vi "Close Module.vi"(8 "error in (no error)":errorcluster, 11 "Module Admin in":refnum<class "Delacor_lib_QMH_Module Admin.lvclass">) -> (0 "error out":errorcluster, 1 "External Launch":bool, 3 "Module Admin out":refnum<class "Delacor_lib_QMH_Module Admin.lvclass">)   [LabVIEW 2020, in "Numpad.lvlib"]
doc: "Destroy the Broadcast Events and Request Events. Reset flags stored in Module Admin class.\n_____\nBased on Delacor QMH Project Template 5.0.0.82."
uses:
  Numpad.lvlib
  <vilib>/Delacor/Delacor QMH/Libraries/Module Admin_class/Delacor_lib_QMH_Module Admin.lvclass
  <vilib>/Delacor/Delacor QMH/Libraries/Module Admin_class/Delacor_lib_QMH_Module Admin.lvclass/Delacor_lib_QMH_Module Admin.ctl
  <vilib>/Delacor/Delacor QMH/Libraries/Module Admin_class/Delacor_lib_QMH_Get External Launch.vi
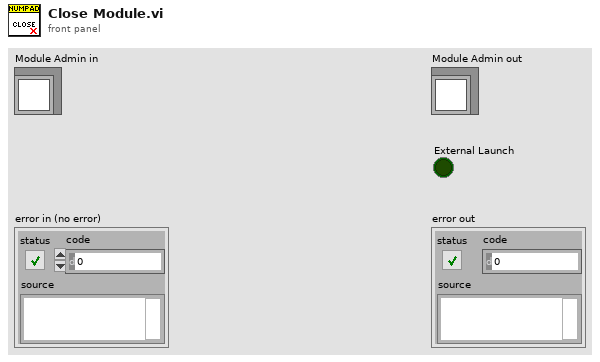
[diagram p1: front panel]
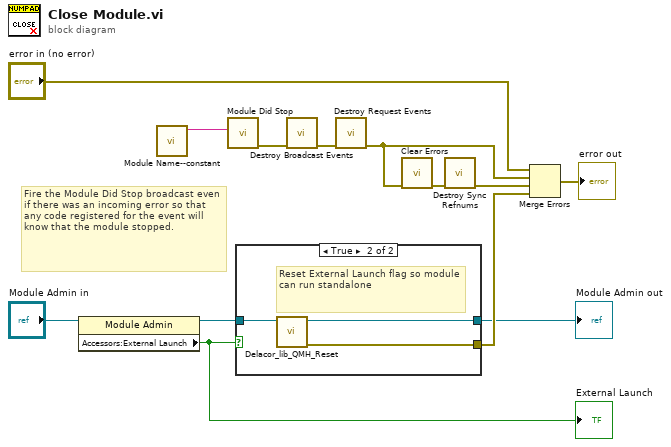
[diagram p0: block diagram]
diagram:
  # "Fire the Module Did Stop broadcast even if there was an incoming error so that any code registered for the event will know that the module stopped."
  n1 = property class="Module Admin"(reference="Module Admin in") -> (reference out=w11:refnum<class "Delacor_lib_QMH_Module Admin.lvclass">, "Accessors:External Launch"=w8:bool)  [unwired: 1 in, 1 out]
  "External Launch" <- w8
  n2 = call "Module Name--constant.vi"() -> ("Module Name"=w6:string)  [unwired: 11 in]
  n3 = call "Module Did Stop.vi"("Origin"=w6) -> ("error out"=w5:errorcluster)  [unwired: 10 in]
  n4 = case shown="True" w8 {
    tunnel: w11 -> [w14 w17]
    tunnel: [w14 w16] -> w9
    tunnel: [_ w15] -> w13
    frame False {
    }
    frame True {
      # "Reset External Launch flag so module can run standalone"
      n5 = call-dynamic "Delacor_lib_QMH_Reset.vi"("Mod Admin in"=w17) -> ("error out"=w15:errorcluster, "Mod Admin out"=w16:refnum<class "Delacor_lib_QMH_Module Admin.lvclass">)  [unwired: 9 in]
    }
  }
  "Module Admin out" <- w9
  n6 = call "Destroy Broadcast Events.vi"("error in (no error)"=w5) -> ("error out"=w7:errorcluster)  [unwired: 10 in]
  n7 = call "Destroy Request Events.vi"("error in (no error)"=w7) -> ("error out"=w12:errorcluster)  [unwired: 10 in]
  n8 = call <vilib>:"Clear Errors.vi"("error in (no error)"=w12) -> ("error out"=w2:errorcluster)  [unwired: 5 in, 1 out]
  n9 = call "Destroy Sync Refnums.vi"("error in (no error)"=w2) -> ("error out"=w4:errorcluster)  [unwired: 10 in]
  n10 = Merge Errors("error in (no error)", w12, w4, w13) -> (→"error out":errorcluster)
